vi "Process State(Initialize).vi"(0 "Process In":refnum<class "Process.lvclass">, 11 "Error In":errorcluster) -> (4 "Process Out":refnum<class "Process.lvclass">, 15 "Error Out":errorcluster)   [LabVIEW 2023, in "Process.lvclass"]
doc: "Method encapsulating Initialize state of process."
uses:
  Process.lvclass
  Interfaces/ICanCommunicate/Message.ctl
  Process.lvclass/Process.ctl
  Interfaces/ICanCommunicate/ICanCommunicate.lvclass
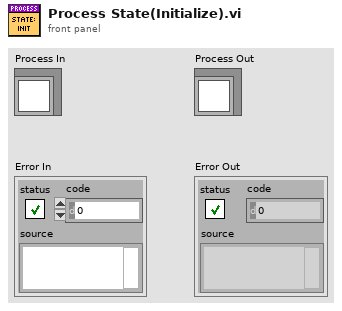
[diagram p1: front panel]
types:
  T1 = typedef "ICanCommunicate.lvclass/Message.ctl" = cluster{"Sender Name":string, "Recipent Name":string, "Command":string, "Data":variant, "Time Stamp":timestamp, "GUID":string, "Chcecksum":string}
  T2 = typedef "ICanCommunicate.lvclass/ProcessSyncQueue.ctl" = refnum<queue>
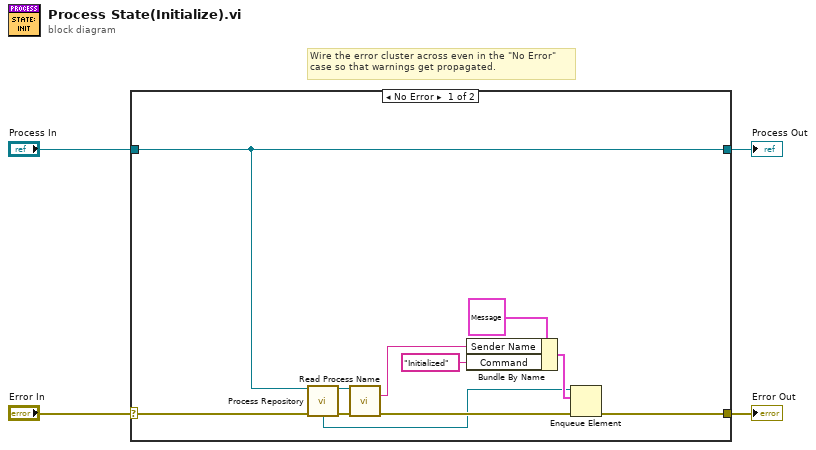
[diagram p0: block diagram]
diagram:
  # "Wire the error cluster across even in the \"No Error\"\ncase so that warnings get propagated."
  n1 = case shown="No Error" "Error In" {
    selector: "Error In" -> [w7 w17]
    tunnel: [w6 w17] -> w3
    tunnel: [w5 w16] -> w1
    tunnel: "Process In" -> [w5 w16]
    frame No Error {
      n2 = call-dynamic "Process Repository.vi"("Process In"=w5, "Error In"=w7) -> ("Process Out"=w14:refnum<class "Process.lvclass">, "ProcessSyncQueue"=w9:T2, "Error Out"=w8:errorcluster)  [unwired: 7 in, 4 out]
      n3 = call "Read Process Name.vi"("Process In"=w14, "Error In"=w8) -> ("Process Name"=w15:string, "Error Out"=w13:errorcluster)  [unwired: 11 in, 1 out]
      n4 = Bundle By Name(cluster=T1 {"Sender Name"="", "Recipent Name"="", "Command"="", "Data"=variant, "Time Stamp"=timestamp(0 s since 1904-01-01), "GUID"="", "Chcecksum"=""} ("element"), "Sender Name"=w15, "Command"="Initialized") -> (w11:T1)
      n5 = Enqueue Element(queue=w9, element=w11, error in (no error)=w13) -> (error out=w6:errorcluster)  [unwired: 1 in, 2 out]
    }
    frame Error {
    }
  }
  "Error Out" <- w3
  "Process Out" <- w1
